vi "PM103 Scope Sample SW Trigger.vi"() -> ()   [LabVIEW 2019]
panel:
  out "TriggerForced":bool
  out "Scope":cluster{"Time Stamps":sgl[], "Values":sgl[]}(graph)
  in  "Autoset":bool
  out "Active":bool
  in  "stop":bool
  # "Thorlabs Power Meter Series\n       PM103 Scope SW Trigger"
  # "This example will connect the first found power meter.\nTo use this sample you need a PM103 with a photodiode sensor."
  # "Connected"
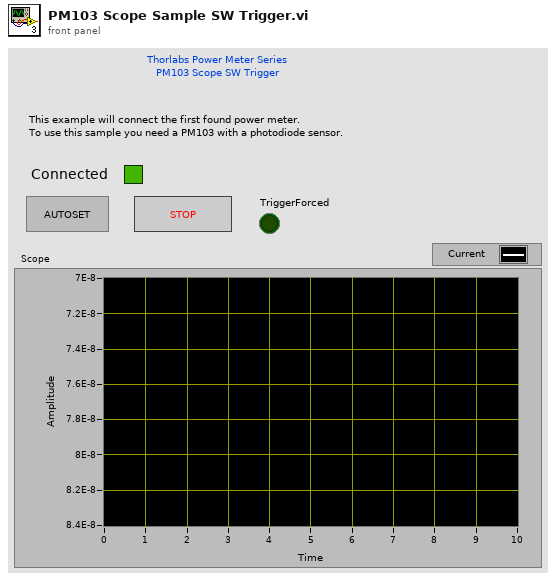
[diagram p1: front panel]
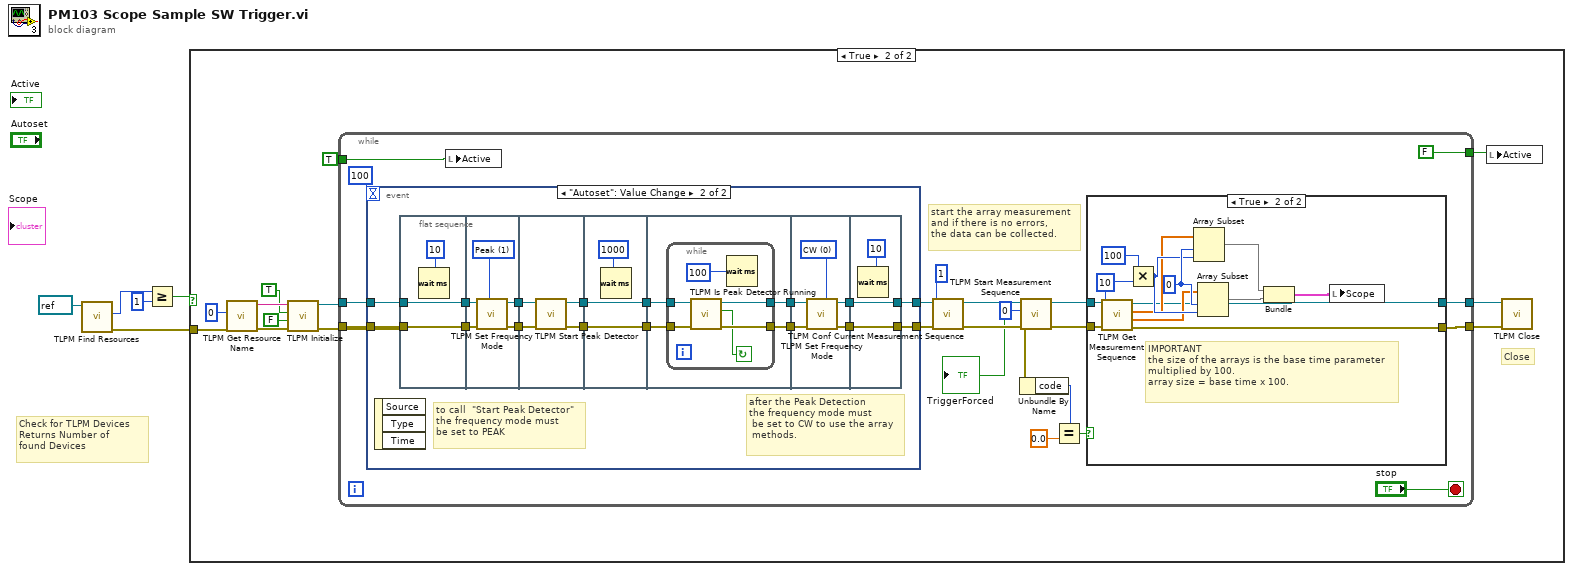
[diagram p0: block diagram]
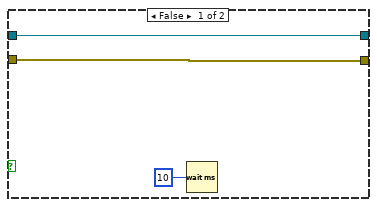
[diagram p3: hidden frame]
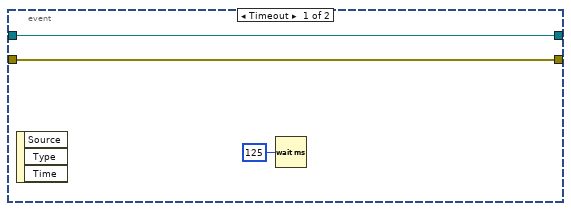
[diagram p4: hidden frame]
diagram:
  # "Check for TLPM Devices\nReturns Number of\nfound Devices"
  n1 = call <instrlib>:"TLPM Find Resources.vi"("instrument handle"=refnum<visa-resource-name> refnum) -> ("error out"=w1:errorcluster, "Resource Count"=w2:u32)  [unwired: 8 in, 1 out]
  n2 = Greater Or Equal?(x=w2, y=u32 1) -> (x >= y?=w3:bool)
  n3 = case shown="True" w3 {
    tunnel: w1 -> [_ w17]
    frame False {
    }
    frame True {
      # "Close"
      n4 = call <instrlib>:"TLPM Get Resource Name.vi"("error in (no error)"=w17, "Index (0)"=u32 0) -> ("error out"=w12:errorcluster, "Resource Name"=w15:string)  [unwired: 7 in, 1 out]
      n5 = call <instrlib>:"TLPM Initialize.vi"("error in (no error)"=w12, "Reset Device (Reset Device)"=FALSE, "ID Query (Do Query)"=TRUE, "resource name"=w15) -> ("error out"=w6:errorcluster, "instrument handle out"=w7:refnum<visa-resource-name>)  [unwired: 6 in]
      n6 = while {
        tunnel: w7 -> [w36]
        tunnel: w6 -> [w35]
        tunnel: [w29] -> w11
        tunnel: [w28] -> w10
        tunnel: TRUE -> [w27]
        tunnel: [FALSE] -> w8
        stop <- "stop" stop-if-true
        # "start the array measurement\nand if there is no errors,\nthe data can be collected."
        n7 = event shown="[1] \"Autoset\": Value Change" {
          selector: _ -> [_ _]
          dyn-events: _ -> [_ _]
          timeout: 100 -> [_ _]
          tunnel: w36 -> [w56 w72]
          tunnel: w35 -> [w55 w71]
          tunnel: [w56 w68] -> w23
          tunnel: [w55 w67] -> w24
          event Timeout {
            n8 = event-data() -> ()  [unwired: 1 in, 3 out]
            n9 = Wait (ms)(milliseconds to wait=u32 125) -> ()  [unwired: 1 out]
          }
          event "Autoset": Value Change {
            # "after the Peak Detection \nthe frequency mode must\n be set to CW to use the array\n methods."
            # "to call  \"Start Peak Detector\"\nthe frequency mode must \nbe set to PEAK"
            n10 = event-data() -> ()  [unwired: 1 in, 3 out]
            n11 = flat-sequence {
              tunnel: w72 -> [w74]
              tunnel: w71 -> [w75]
              tunnel: [w74] -> w62
              tunnel: [w75] -> w60
              tunnel: w62 -> [w76]
              tunnel: [w77] -> w61
              tunnel: w60 -> [w79]
              tunnel: [w78] -> w59
              tunnel: w61 -> [w84]
              tunnel: w59 -> [w83]
              tunnel: [w82] -> w66
              tunnel: [w81] -> w64
              tunnel: w66 -> [w87]
              tunnel: [w87] -> w65
              tunnel: w64 -> [w86]
              tunnel: [w86] -> w63
              tunnel: w65 -> [w90]
              tunnel: w63 -> [w91]
              tunnel: [w89] -> w70
              tunnel: [w88] -> w69
              tunnel: w70 -> [w101]
              tunnel: w69 -> [w100]
              tunnel: [w99] -> w58
              tunnel: [w98] -> w57
              tunnel: [w104] -> w68
              tunnel: [w105] -> w67
              tunnel: w58 -> [w105]
              tunnel: w57 -> [w104]
              frame #0 {
                n12 = Wait (ms)(milliseconds to wait=u32 10) -> ()  [unwired: 1 out]
              }
              frame #1 {
                w80 = u16 1 items=["CW", "Peak"] ("Frequency Mode (Peak)")
                n13 = call <instrlib>:"TLPM Set Frequency Mode.vi"("error in (no error)"=w79, "Frequency Mode (Peak)"=w80, "instrument handle"=w76) -> ("error out"=w78:errorcluster, "instrument handle out"=w77:refnum<visa-resource-name>)  [unwired: 7 in]
              }
              frame #2 {
                n14 = call <instrlib>:"TLPM Start Peak Detector.vi"("error in (no error)"=w83, "instrument handle"=w84) -> ("error out"=w82:errorcluster, "instrument handle out"=w81:refnum<visa-resource-name>)  [unwired: 8 in]
              }
              frame #3 {
                n15 = Wait (ms)(milliseconds to wait=u32 1000) -> ()  [unwired: 1 out]
              }
              frame #4 {
                n16 = while {
                  tunnel: w91 -> [w96]
                  tunnel: w90 -> [w95]
                  tunnel: [w94] -> w88
                  tunnel: [w93] -> w89
                  stop <- w92 continue-if-true
                  n17 = call <instrlib>:"TLPM Is Peak Detector Running.vi"("error in (no error)"=w95, "instrument handle"=w96) -> ("error out"=w94:errorcluster, "Is Running"=w92:bool, "instrument handle out"=w93:refnum<visa-resource-name>)  [unwired: 7 in]
                  n18 = Wait (ms)(milliseconds to wait=u32 100) -> ()  [unwired: 1 out]
                }
              }
              frame #5 {
                w102 = u16 0 items=["CW", "Peak"] ("Frequency Mode (Peak)")
                n19 = call <instrlib>:"TLPM Set Frequency Mode.vi"("error in (no error)"=w100, "Frequency Mode (Peak)"=w102, "instrument handle"=w101) -> ("error out"=w99:errorcluster, "instrument handle out"=w98:refnum<visa-resource-name>)  [unwired: 7 in]
              }
              frame #6 {
                n20 = Wait (ms)(milliseconds to wait=u32 10) -> ()  [unwired: 1 out]
              }
            }
          }
        }
        n21 = local write "Active"(w27) -> ()
        n22 = call <instrlib>:"TLPM Conf Current Measurement Sequence.vi"("error in (no error)"=w24, "Averaging Limit"=u32 1, "instrument handle"=w23) -> ("error out"=w21:errorcluster, "instrument handle out"=w22:refnum<visa-resource-name>)  [unwired: 7 in]
        n23 = call <instrlib>:"TLPM Start Measurement Sequence.vi"("error in (no error)"=w21, "AutoTriggerDelay (0)"=u32 0, "instrument handle"=w22) -> ("error out"=w31:errorcluster, "TriggerForced"=→"TriggerForced":bool, "instrument handle out"=w34:refnum<visa-resource-name>)  [unwired: 6 in]
        n24 = Unbundle By Name(w31) -> ("code"=w30:i32)
        n25 = Equal?(x=w30, y=0.0) -> (x = y?=w33:bool)
        n26 = case shown="True" w33 {
          tunnel: w31 -> [w39 w46]
          tunnel: w34 -> [w40 w47]
          tunnel: [w39 w45] -> w28
          tunnel: [w40 w42] -> w29
          frame False {
            n27 = Wait (ms)(milliseconds to wait=u32 10) -> ()  [unwired: 1 out]
          }
          frame True {
            w52 = 0 ("index")
            w41 = u32 10 ("Base Time")
            # "IMPORTANT\nthe size of the arrays is the base time parameter\nmultiplied by 100.\narray size = base time x 100."
            n28 = call <instrlib>:"TLPM Get Measurement Sequence.vi"("error in (no error)"=w46, "Base Time"=w41, "instrument handle"=w47) -> ("error out"=w45:errorcluster, "Values"=w44:sgl[], "Time Stamps"=w43:sgl[], "instrument handle out"=w42:refnum<visa-resource-name>)  [unwired: 5 in]
            n29 = Multiply(x=u32 100, y=w41) -> (x*y=w51:u32)
            n30 = Array Subset(array=w43, index=w52, length=w51) -> (w50:sgl[])
            n31 = Array Subset(array=w44, index=w52, length=w51) -> (w49:sgl[])
            n32 = Bundle(w50, w49) -> (w48:cluster{sgl[], sgl[]})  [unwired: 1 in]
            n33 = local write "Scope"(w48) -> ()
          }
        }
      }
      n34 = local write "Active"(w8) -> ()
      n35 = call <instrlib>:"TLPM Close.vi"("error in (no error)"=w10, "instrument handle"=w11) -> ()  [unwired: 9 in, 1 out]
    }
  }
